vi "Database-SQLiteStorePlugConn.vi"(8 "error in (no error)":errorcluster, 9 "ActorID":string, 10 "FTW Actor Connector":refnum<class "FTW-ActorConnector.lvclass">, 11 "Database-Actor in":refnum<class "Database-Actor.lvclass">) -> (0 "error out":errorcluster, 3 "Database-Actor out":refnum<class "Database-Actor.lvclass">)   [LabVIEW 2013, in "Database-Actor.lvclass"]
uses:
  Database-Actor.lvclass
  ftw-dataflow/Actor/src/Connector/FTW-ActorConnector.lvclass
  Database-Actor.lvclass/Database-Actor.ctl
  ftw-dataflow/Core/src/Database/FTW-SQLite-Connector.lvclass
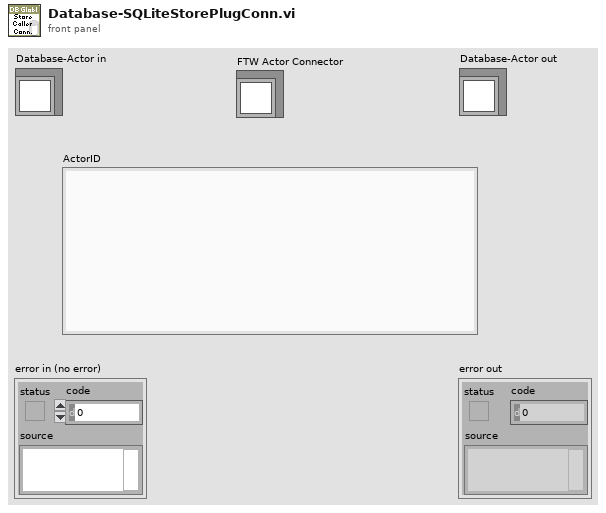
[diagram p1: front panel]
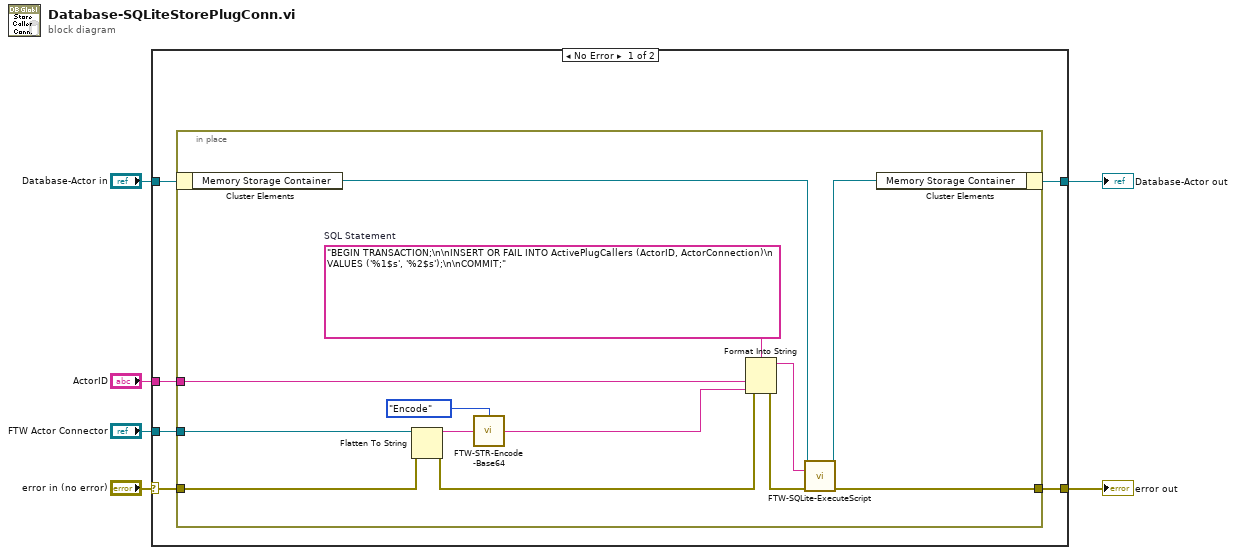
[diagram p0: block diagram]
diagram:
  n1 = case shown="No Error" "error in (no error)" {
    selector: "error in (no error)" -> [w10 w27]
    tunnel: [w7 w27] -> w5
    tunnel: [w8 w26] -> w3
    tunnel: "Database-Actor in" -> [w9 w26]
    tunnel: "ActorID" -> [w12 _]
    tunnel: "FTW Actor Connector" -> [w11 _]
    frame No Error {
      n2 = in-place {
        in-place-border: [w23] -> w7
        in-place-border: w10 -> [w15]
        in-place-border: w11 -> [w20]
        in-place-border: w12 -> [w16]
        w24 = "BEGIN TRANSACTION;\n\nINSERT OR FAIL INTO ActivePlugCallers (ActorID, ActorConnection)\n    VALUES ('%1$s', '%2$s');\n\nCOMMIT;"  # SQL Statement
        n3 = in-place-cluster #1(w9) -> ("Memory Storage Container"=w21:refnum<class "FTW-SQLite-Connector.lvclass">)
        n4 = Flatten To String(anything=w20, error in (no error)=w15) -> (data string=w19:string, error out=w14:errorcluster)  [unwired: 2 in, 1 out]
        n5 = call "FTW-STR-Encode-Base64.vi"("Input"=w19, "Direction"=enum16{"Encode", "Decode"}."Encode") -> ("Output"=w17:string)
        n6 = Format Into String(format string=w24, error in=w14, w16, w17) -> (resulting string=w25:string, error out=w13:errorcluster)  [unwired: 1 in]
        n7 = call "FTW-SQLite-ExecuteScript.vi"("SQLite Connector"=w21, "SQL Script"=w25, "error in"=w13) -> ("SQLite Connector out"=w22:refnum<class "FTW-SQLite-Connector.lvclass">, "error out"=w23:errorcluster)  [unwired: 9 in, 2 out]
        n8 = in-place-cluster #1("Memory Storage Container"=w22) -> (w8:refnum<class "Database-Actor.lvclass">)
      }
    }
    frame Error {
    }
  }
  "error out" <- w5
  "Database-Actor out" <- w3
